vi "Test Coffee Shop Cashier Order Items Sent to Order Queue.vi"(8 "error in (no error)":errorcluster, 11 "Coffee Shop Test in":refnum<class "Coffee Shop Test.lvclass">) -> (0 "error out":errorcluster, 3 "Coffee Shop Test out":refnum<class "Coffee Shop Test.lvclass">)   [LabVIEW 2020, in "Coffee Shop Test.lvclass"]
uses:
  Coffee Shop Test.lvclass
  C:/Program Files (x86)/National Instruments/LabVIEW 2020/vi.lib/Asteme/LUnit/Test Case.lvclass
  Coffee Shop/Coffee Shop.lvclass
  C:/Program Files (x86)/National Instruments/LabVIEW 2020/vi.lib/Asteme/Triarc Framework/Process/Process.lvclass
  C:/Program Files (x86)/National Instruments/LabVIEW 2020/vi.lib/Asteme/Triarc Framework/Application/Application.lvclass
  Mock Worker/Mock Job Handler.lvclass
  C:/Users/anton/Documents/GitHub/Triarc-Examples/Coffee Shop/Process Job/Job Handler.lvclass
  Cashier/Cashier.lvclass
  Support/Beverages/TypeDefs/Drink Type.ctl
  Support/Beverages/TypeDefs/Options.ctl
  Customer/Customer.lvclass
  <vilib>/Asteme/Triarc Framework/Process/Process.lvclass/Process.ctl
  <vilib>/Asteme/Triarc Framework/Application/Application.lvclass/Application.ctl
  <vilib>/Asteme/LUnit/Test Case.lvclass/Test Case.ctl
  <vilib>/Asteme/LUnit/LUnit Assertion Result.lvclass/LUnit Assertion Result.ctl
  <vilib>/Asteme/Triarc Framework/Process/Public/Lifecycle/Get Lifecycle State.vi
  <vilib>/Asteme/Triarc Framework/Process/Protected/Messaging/Request Message.vi
  <vilib>/Asteme/Triarc Framework/Process/Private/SubVIs/Wait for finish.vi
  <vilib>/Asteme/Triarc Framework/Process/Protected/Messaging/Enqueue Message.vi
  <vilib>/Asteme/Triarc Framework/Process/Private/SubVIs/Set Lifecycle State.vi
  <vilib>/Asteme/LUnit/Palette/Pass If.vi
  <vilib>/Asteme/LUnit/Set Assertion Type.vi
  <vilib>/Utility/error.llb/Clear Errors.vi
  <vilib>/Asteme/Triarc Framework/Process/Private/SubVIs/Enqueue Request Message.vi
  <vilib>/AdvancedString/1D String Array to Delimited String.vi
  <vilib>/Asteme/LUnit/Palette/Fail.vi
  <vilib>/Asteme/LUnit/Palette/Pass.vi
  <vilib>/Asteme/LUnit/LUnit Write Assertion Type.vi
  <vilib>/Asteme/LUnit/Add test result.vi
  <vilib>/Asteme/LUnit/LUnit Write Passed.vi
  <vilib>/Asteme/LUnit/LUnit Get Test Case.vi
  <vilib>/Asteme/LUnit/Assertion Result/LUnit Get Test Name.vi
  <vilib>/Asteme/LUnit/LUnit Write Message.vi
  <vilib>/Asteme/LUnit/LUnit Write Description.vi
  <vilib>/Asteme/LUnit/Read Test Case Name.vi
  <vilib>/Asteme/Triarc Framework/Application/Application.lvclass
  <vilib>/Utility/error.llb/Error Cluster From Error Code.vi
  <vilib>/Asteme/Triarc Framework/Process/Private/SubVIs/Wait for Response Message.vi
  <vilib>/Asteme/Triarc Framework/Process/Process.lvclass
  <vilib>/Asteme/LUnit/LUnit Assertion Result.lvclass
  C:/Program Files (x86)/National Instruments/LabVIEW 2020/vi.lib/Asteme/Triarc Framework/Base/Base.lvclass
  C:/Program Files (x86)/National Instruments/LabVIEW 2020/vi.lib/Asteme/Triarc Framework/Error Handler Interface/Error Handler Interface.lvclass
  C:/Program Files (x86)/National Instruments/LabVIEW 2020/vi.lib/Asteme/Triarc Framework/Logging/Logging.lvclass
  C:/Users/anton/Documents/GitHub/Triarc-Examples/Coffee Shop/Coffee Shop/Coffee Shop.lvclass
  Support/Beverages/Beverage/Beverage.lvclass
  <vilib>/Asteme/LUnit/Test Case.lvclass
  Support/Order/Order.lvclass
  C:/Users/anton/Documents/GitHub/Triarc-Examples/Coffee Shop/Mock Worker/Mock Job Handler.lvclass
  C:/Program Files (x86)/National Instruments/LabVIEW 2020/vi.lib/Asteme/Triarc Framework Test Suite/Application Test/Application Test.lvclass
  C:/Program Files (x86)/National Instruments/LabVIEW 2020/vi.lib/Asteme/Triarc Framework Test Suite/Process Test/Process Test.lvclass
  C:/Program Files (x86)/National Instruments/LabVIEW 2020/vi.lib/Asteme/Triarc Framework Test Suite/Base Class Test/Base Test.lvclass
  C:/Users/anton/Documents/GitHub/Triarc-Examples/Coffee Shop/Coffee Shop Test/Coffee Shop Test.lvclass
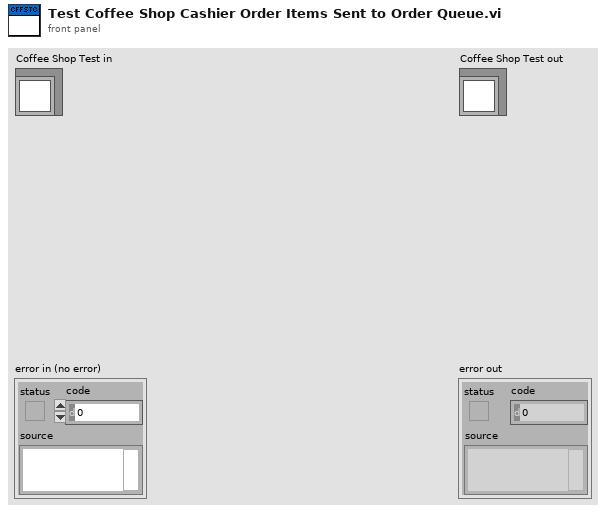
[diagram p1: front panel]
types:
  T1 = typedef "Beverage.lvclass/Drink Type.ctl" = enum16{"Dark Roast", "Decaf", "Espresso", "House Blend"}
  T2 = typedef "Beverage.lvclass/Options.ctl" = enum16{"<None>", "Milk", "Mocha", "Soy", "Whip"}
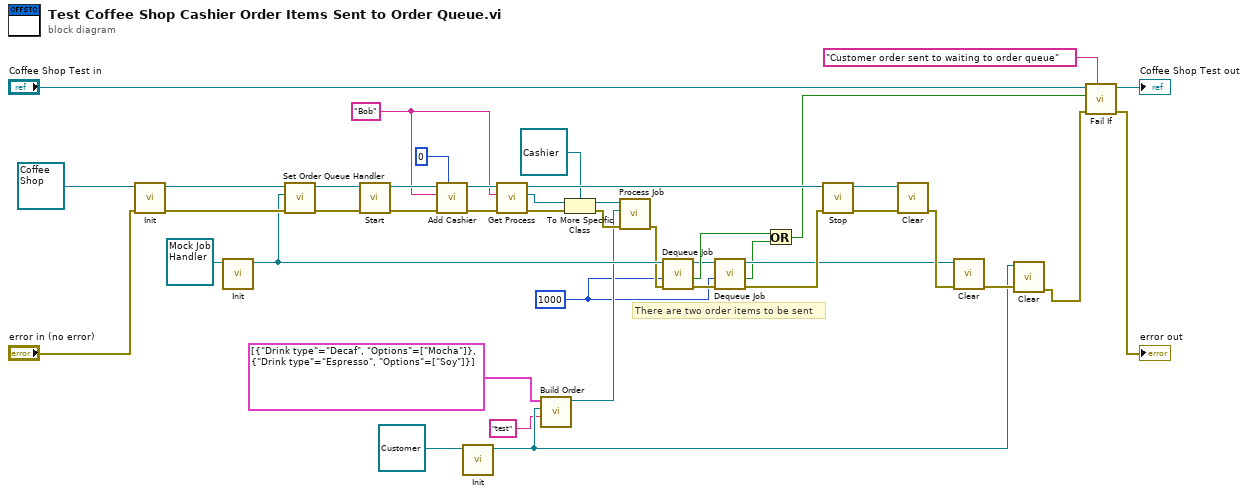
[diagram p0: block diagram]
diagram:
  w4 = 1000 ("timeout in ms (-1)")
  w21 = "Bob" ("Name")
  # "There are two order items to be sent"
  n1 = call-dynamic "Init.vi"("error in (no error)"="error in (no error)", "Process In"=refnum<class "Coffee Shop.lvclass"> refnum ("Coffee Shop.lvclass")) -> ("error out"=w43:errorcluster, "Process Out"=w36:refnum<class "Coffee Shop.lvclass">)  [unwired: 8 in]
  n2 = call-dynamic "Init.vi"("Mock Job Handler In"=refnum<class "Mock Job Handler.lvclass"> refnum) -> ("Mock Job Handler Out"=w31:refnum<class "Mock Job Handler.lvclass">)  [unwired: 9 in, 1 out]
  n3 = call "Set Order Queue Handler.vi"("error in (no error)"=w43, "Order Queue Handler"=w31, "Coffee Shop In"=w36) -> ("error out"=w41:errorcluster, "Coffee Shop Out"=w42:refnum<class "Coffee Shop.lvclass">)  [unwired: 7 in]
  n4 = call <vilib>:"Start.vi"("error in (no error)"=w41, "Process In"=w42) -> ("error out"=w40:errorcluster, "Process Out"=w35:refnum<class "Coffee Shop.lvclass">)  [unwired: 8 in]
  n5 = call "Add Cashier.vi"("Time Scale [ms]"=u32 0, "error in (no error)"=w40, "Name"=w21, "Coffee Shop in"=w35) -> ("error out"=w33:errorcluster, "Coffee Shop out"=w23:refnum<class "Coffee Shop.lvclass">)  [unwired: 6 in]
  n6 = call-dynamic "Init.vi"("View In"=refnum<class "Customer.lvclass"> refnum ("Customer.lvclass")) -> ("View Out"=w10:refnum<class "Customer.lvclass">)  [unwired: 9 in, 1 out]
  n7 = call <vilib>:"Get Process.vi"("error in (no error)"=w33, "Process Name"=w21, "Rig In"=w23) -> ("error out"=w24:errorcluster, "App Process"=w20:refnum<class "Process.lvclass">, "Rig Out"=w22:refnum<class "Coffee Shop.lvclass">)  [unwired: 6 in]
  n8 = call "Build Order.vi"("Customer Name"="test", "Customer"=w10, "Order"=cluster{"Drink type":T1, "Options":T2[]}[] [{"Drink type"=enum."Decaf", "Options"=[enum."Mocha"]}, {"Drink type"=enum."Espresso", "Options"=[enum."Soy"]}] ("Order Content")) -> ("Order Out"=w8:refnum<class "Order.lvclass">)  [unwired: 7 in, 1 out]
  n9 = To More Specific Class(target class=refnum<class "Cashier.lvclass"> refnum ("Cashier.lvclass"), reference=w20, error in=w24) -> (specific class reference=w15:refnum<class "Cashier.lvclass">, error out=w16:errorcluster)
  n10 = call-dynamic "Process Job.vi"("error in (no error)"=w16, "Job"=w8, "Worker In"=w15) -> ("error out"=w18:errorcluster)  [unwired: 7 in, 1 out]
  n11 = call "Dequeue Job.vi"("error in (no error)"=w18, "timeout in ms (-1)"=w4, "Mock Job Handler In"=w31) -> ("error out"=w26:errorcluster, "timed out?"=w17:bool, "Mock Job Handler Out"=w6:refnum<class "Mock Job Handler.lvclass">)  [unwired: 5 in, 1 out]
  n12 = call "Dequeue Job.vi"("error in (no error)"=w26, "timeout in ms (-1)"=w4, "Mock Job Handler In"=w6) -> ("error out"=w7:errorcluster, "timed out?"=w2:bool, "Mock Job Handler Out"=w5:refnum<class "Mock Job Handler.lvclass">)  [unwired: 5 in, 1 out]
  n13 = Or(x=w17, y=w2) -> (x .or. y?=w3:bool)
  n14 = call <vilib>:"Stop.vi"("error in (no error)"=w7, "Process In"=w22) -> ("error out"=w38:errorcluster, "Process Out"=w39:refnum<class "Coffee Shop.lvclass">)  [unwired: 7 in, 1 out]
  n15 = call-dynamic "Clear.vi"("error in (no error)"=w38, "Application In"=w39) -> ("error out"=w32:errorcluster)  [unwired: 9 in]
  n16 = call-dynamic "Clear.vi"("error in (no error)"=w32, "Mock Job Handler In"=w5) -> ("error out"=w12:errorcluster)  [unwired: 9 in]
  n17 = call-dynamic "Clear.vi"("error in (no error)"=w12, "View In"=w10) -> ("error out"=w11:errorcluster)  [unwired: 9 in]
  n18 = call <vilib>:"Fail If.vi"("Description"="Customer order sent to waiting to order queue", "error in (no error)"=w11, "Fail?"=w3, "Test Case In"="Coffee Shop Test in") -> ("error out"=→"error out":errorcluster, "Test Case Out"=→"Coffee Shop Test out":refnum<class "Coffee Shop Test.lvclass">)  [unwired: 6 in]
